vi "ArrayDemo.vi"() -> ()   [LabVIEW 2018]
panel:
  out "Array Size":dbl
  out "Minimum Value":dbl
  out "Minimum Value Index":dbl
  out "Maximum Value Index":dbl
  out "Maximum Value":dbl
  in  "?":bool
  in  "OK Button":bool
  in  "Maximum Value":dbl=100.0
  in  "Minimum Value":dbl
  in  "Number of Array Elements":dbl=1000.0
  out "Array":dbl[](array[numeric])
  # "Integers Only"
  # "Real Numbers"
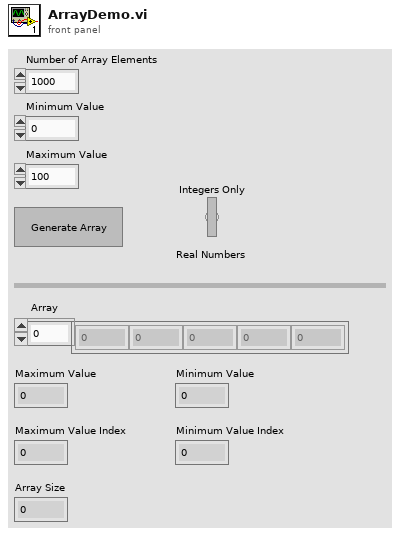
[diagram p1: front panel]
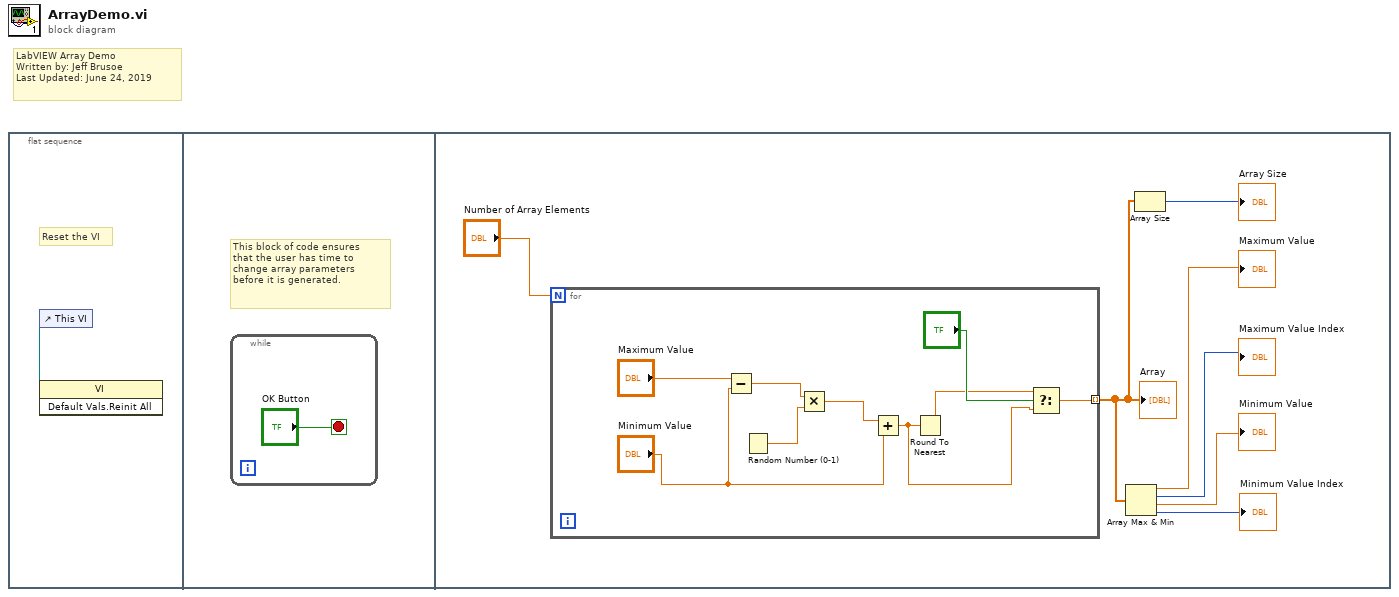
[diagram p0: block diagram]
diagram:
  # "LabVIEW Array Demo\nWritten by: Jeff Brusoe\nLast Updated: June 24, 2019"
  n1 = flat-sequence {
    frame #0 {
      # "Reset the VI"
      n2 = control-ref of="This VI"() -> (w1:refnum<vi>)
      n3 = invoke class="VI" method="Default Vals.Reinit All"(reference=w1) -> ()  [unwired: 2 in, 3 out]
    }
    frame #1 {
      # "This block of code ensures\nthat the user has time to \nchange array parameters\nbefore it is generated."
      n4 = while {
        stop <- "OK Button" stop-if-true
      }
    }
    frame #2 {
      n5 = for {
        N: "Number of Array Elements" -> [_]
        tunnel: [w10] -> w3 mode=indexing
        n6 = Subtract(x="Maximum Value", y="Minimum Value") -> (x-y=w14:dbl)
        n7 = Random Number (0-1)() -> (number: 0 to 1=w17:dbl)
        n8 = Multiply(x=w14, y=w17) -> (x*y=w16:dbl)
        n9 = Add(x=w16, y="Minimum Value") -> (x+y=w11:dbl)
        n10 = Round To Nearest(number=w11) -> (nearest integer value=w12:dbl)
        n11 = Select(t=w12, s="?", f=w11) -> (s? t:f=w10:dbl)
      }
      "Array" <- w3
      n12 = Array Max & Min(array=w3) -> (max value=→"Maximum Value":dbl, max index (indices)=→"Maximum Value Index":i32, min value=→"Minimum Value":dbl, min index (indices)=→"Minimum Value Index":i32)
      n13 = Array Size(array=w3) -> (size(s)=→"Array Size":i32)
    }
  }
